vi "Redim.vi"(8 "error in":errorcluster, 9 "Columns":i32, 10 "Rows":i32, 11 "Sourcegrid in":refnum<class "SourceGrid.lvclass">) -> (0 "error out":errorcluster, 3 "Sourcegrid out":refnum<class "SourceGrid.lvclass">)   [LabVIEW 2024, in "SourceGrid.lvlib" / "SourceGrid.lvclass"]
doc: "Set the number of columns and rows"
uses:
  SourceGrid.lvclass
  SourceGrid.lvclass/SourceGrid.ctl
  D:/git/Sourcegrid-LabVIEW/dll/SourceGrid.dll
  dll/SourceGrid.dll
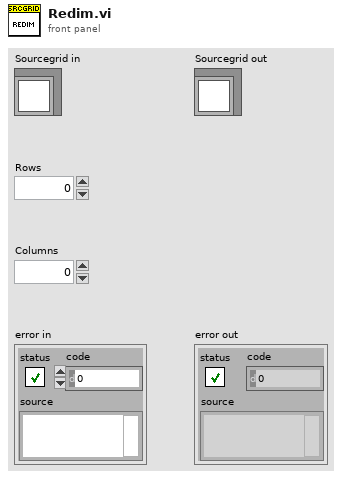
[diagram p1: front panel]
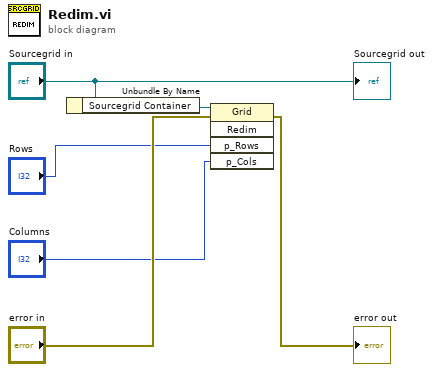
[diagram p0: block diagram]
diagram:
  n1 = Unbundle By Name("Sourcegrid in") -> ("Sourcegrid Container"=w5:refnum<k24>)
  n2 = invoke class="Grid" method="Redim"(reference=w5, error in="error in", "p_Rows"="Rows", "p_Cols"="Columns") -> (error out=→"error out":errorcluster)  [unwired: 1 in, 4 out]
  "Sourcegrid out" <- "Sourcegrid in"
